vi "KML-Create.vi"(5 "path to vi or exe install\\data\\ dir":path) -> (0 "error out":errorcluster)   [LabVIEW 8.6]
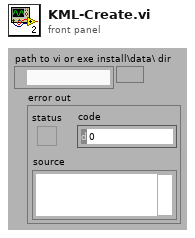
[diagram p1: front panel]
types:
  T1 = enum16{"open", "replace", "create", "open or create", "replace or create", "replace or create with confirmation"}
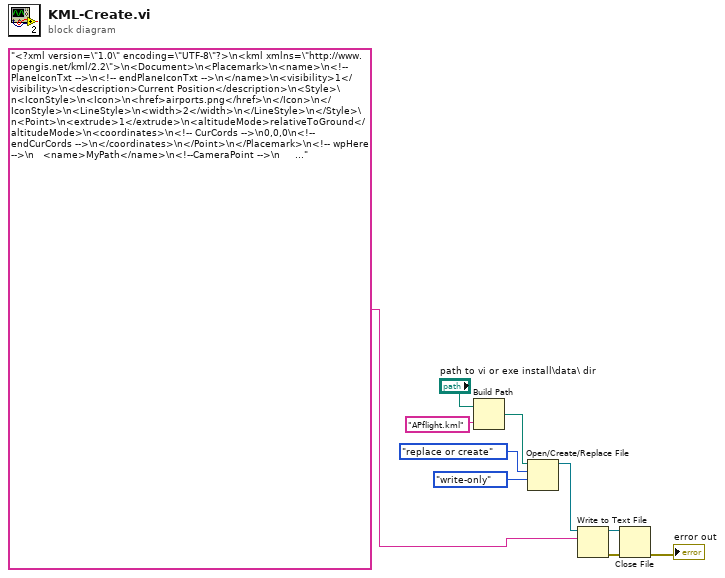
[diagram p0: block diagram]
diagram:
  n1 = Build Path(base path="path to vi or exe install\\data\\ dir", name or relative path="APflight.kml") -> (appended path=w4:path)
  n2 = Open/Create/Replace File(file path (use dialog)=w4, operation (0:open)=T1."replace or create", access (0:read/write)=enum16{"read/write", "read-only", "write-only"}."write-only") -> (refnum out=w7:refnum<file>)  [unwired: 3 in, 2 out]
  n3 = Write to Text File(file (use dialog)=w7, text="<?xml version=\"1.0\" encoding=\"UTF-8\"?>\n<kml xmlns=\"http://www.opengis.net/kml/2.2\">\n<Document>\n<Placemark>\n<name>\n<!-- PlaneIconTxt -->\n<!-- endPlaneIconTxt -->\n</name>\n<visibility>1</visibility>\n<description>Current Position</description>\n<Style>\n<IconStyle>\n<Icon>\n<href>airports.png</href>\n</Icon>\n</IconStyle>\n<LineStyle>\n<width>2</width>\n</LineStyle>\n</Style>\n<Point>\n<extrude>1</extrude>\n<altitudeMode>relativeToGround</altitudeMode>\n<coordinates>\n<!-- CurCords -->\n0,0,0\n<!-- endCurCords -->\n</coordinates>\n</Point>\n</Placemark>\n<!-- wpHere -->\n   <name>MyPath</name>\n<!--CameraPoint -->\n     <LookAt>\n      <longitude>0</longitude>\n      <latitude>0</latitude>  \n      <altitude>0</altitude>  \n       <range>1000</range>   \n      <tilt>0</tilt> \n      <heading>0</heading> \n      <altitudeMode>relativeToGround</altitudeMode>\n    </LookAt>\n<!--endCameraPoint -->\n    <description>Path flown by the plane.</description>\n    <Style id=\"yellowLineGreenPoly\">\n      <LineStyle>\n        <color>7f00ffff</color>\n        <width>4</width>\n      </LineStyle>\n      <PolyStyle>\n        <color>7f00ff00</color>\n      </PolyStyle>\n    </Style>\n    <Placemark>\n      <name>Absolute Extruded</name>\n      <description>Airplane paths</description>\n      <styleUrl>#yellowLineGreenPoly</styleUrl>\n      <LineString>\n        <extrude>1</extrude>\n        <tessellate>1</tessellate>\n        <altitudeMode>relativeToGround</altitudeMode>\n        <coordinates>\n\t<!-- CordPathData -->\n          </coordinates>\n      </LineString>\n    </Placemark>\n  </Document>\n</kml>") -> (refnum out=w8:refnum<file>, error out=w2:errorcluster)  [unwired: 1 in, 2 out]
  n4 = Close File(refnum=w8, error in=w2) -> (error out=→"error out":errorcluster)  [unwired: 1 out]
